vi "異常處理.vi"(7 "VI in":refnum<vi>, 8 "Error In":bool, 9 "Error Array In":i32[](array[numeric]), 10 "AllRef":T1) -> (0 "Error Out":bool, 1 "Error Array Out":i32[](array[numeric]))   [LabVIEW 2015]
uses:
  0.GUI/Control/AllRef.ctl
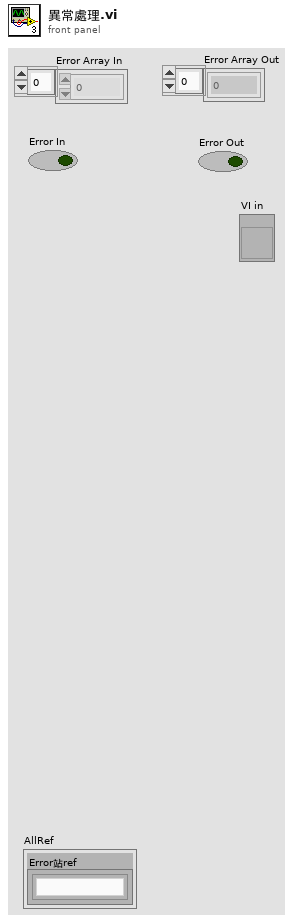
[diagram p1: front panel]
types:
  T1 = typedef "AllRef.ctl" = cluster{"Error站ref":T2}
  T2 = typedef "Error站_ref.ctl" = refnum<k1>
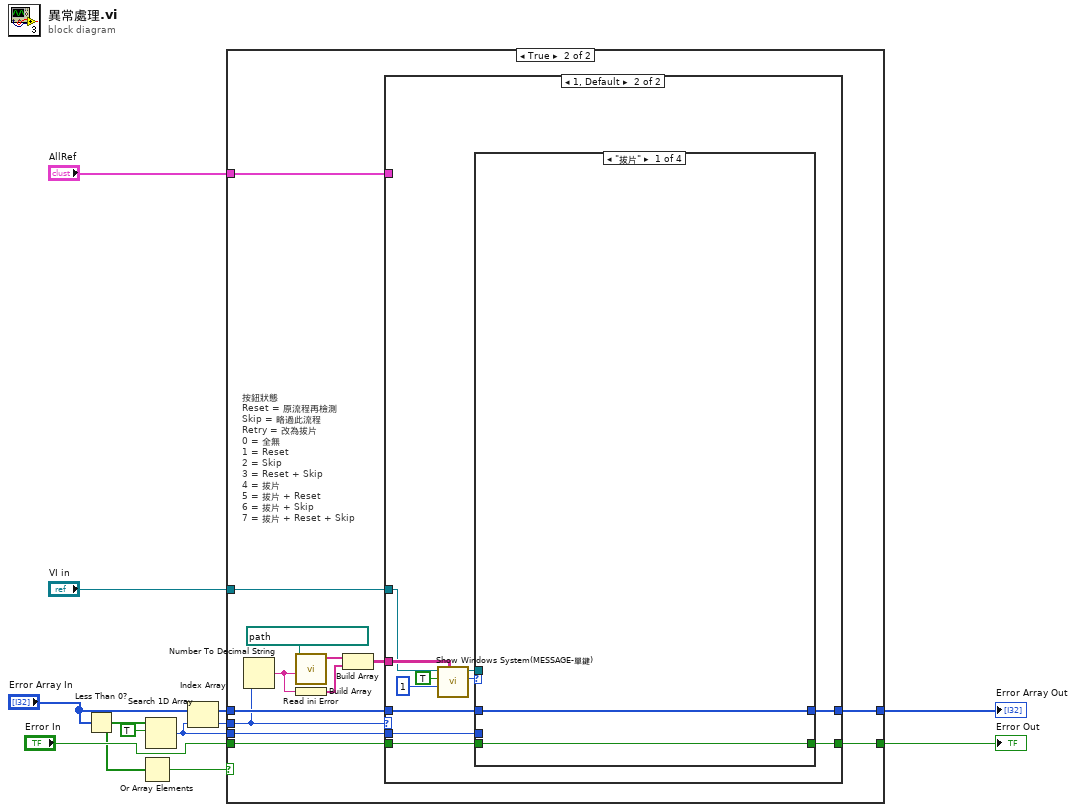
[diagram p0: block diagram]
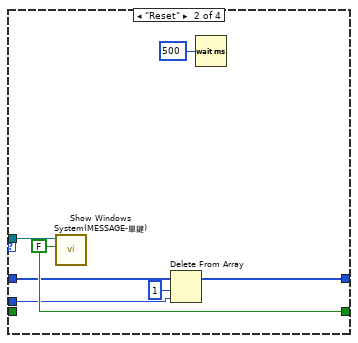
[diagram p4: hidden frame]
diagram:
  n1 = Less Than 0?(x="Error Array In") -> (x < 0?=w2:bool[])
  n2 = Or Array Elements(Boolean array=w2) -> (logical OR=w3:bool)
  n3 = Search 1D Array(1D array=w2, element=TRUE) -> (index of element=w8:i32)  [unwired: 1 in]
  n4 = Index Array(array="Error Array In", index=w8) -> (element=w7:i32)
  n5 = case shown="True" w3 {
    selector: w3 -> [w12 _]
    tunnel: [w13 w23] -> w4
    tunnel: "Error Array In" -> [w13 w25]
    tunnel: [w12 w26] -> w6
    tunnel: w7 -> [_ w18]
    tunnel: w8 -> [_ w24]
    tunnel: "Error In" -> [_ w22]
    tunnel: "VI in" -> [_ w16]
    tunnel: "AllRef" -> [_ w14]
    frame False {
    }
    frame True {
      # "按鈕狀態\nReset = 原流程再檢測\nSkip = 略過此流程\nRetry = 改為拔片\n0 = 全無\n1 = Reset\n2 = Skip\n3 = Reset + Skip\n4 = 拔片\n5 = 拔片 + Reset\n6 = 拔片 + Skip\n7 = 拔片 + Reset + Skip"
      n6 = Number To Decimal String(number=w18) -> (decimal integer string=w20:string)  [unwired: 1 in]
      n7 = call "Read ini Error.vi"("Error Code"=w20, "Error Code file path"=path "D:/半自動電檢機 Data/Error Code.ini") -> ("Error message"=w19:string[])  [unwired: 9 in]
      n8 = Build Array(w20) -> (w21:string[])
      n9 = Build Array(w19, w21) -> (w17:string[][])
      n10 = case shown="1, Default" w18 {
        tunnel: [w27 w36] -> w26
        tunnel: w25 -> [w28 w35]
        tunnel: w24 -> [_ w34]
        tunnel: [w28 w33] -> w23
        tunnel: w22 -> [w27 w32]
        tunnel: w17 -> [_ w31]
        tunnel: w16 -> [_ w29]
        tunnel: w14 -> [_ _]
        frame 0 {
        }
        frame 1, Default {
          n11 = call "Show Windows System(MESSAGE-單鍵).vi"("Error Message Array"=w31, "按鈕狀態"=u8 1, "Show"=TRUE, "vi reference in"=w29) -> ("Selection Result"=w38:enum16{"拔片", "Reset", "Skip", "Nothing"}, "vi reference out"=w37:refnum<vi>)  [unwired: 4 in, 1 out]
          n12 = case shown="\"拔片\"" w38 {
            tunnel: w37 -> [_ w48 _ _]
            tunnel: [w40 w47 w49 w51] -> w36
            tunnel: w35 -> [w41 w45 w50 w52]
            tunnel: w34 -> [_ w44 _ _]
            tunnel: [w41 w43 w50 w52] -> w33
            tunnel: w32 -> [w40 _ w49 w51]
            frame "拔片" {
            }
            frame "Reset" {
              w47 = FALSE ("Show")
              n13 = call "Show Windows System(MESSAGE-單鍵).vi"("Show"=w47, "vi reference in"=w48) -> ()  [unwired: 6 in, 3 out]
              n14 = Delete From Array(array=w45, length=1, index=w44) -> (array with subset deleted=w43:i32[])  [unwired: 1 out]
              n15 = Wait (ms)(milliseconds to wait=u32 500) -> ()  [unwired: 1 out]
            }
            frame "Skip" {
            }
            frame "Nothing", Default {
            }
          }
        }
      }
    }
  }
  "Error Out" <- w6
  "Error Array Out" <- w4
